vi "reinitialize pico.vi"(8 "error in (no error)":errorcluster, 11 "Picomotor8742dotNet in":refnum<class "Picomotor8742dotNet.lvclass">) -> (0 "error out":errorcluster, 2 "new command":string, 3 "Picomotor8742dotNet out":refnum<class "Picomotor8742dotNet.lvclass">)   [LabVIEW 2020, in "Picomotor8742dotNet.lvclass"]
uses:
  Picomotor8742dotNet.lvclass
  Picomotor8742dotNet.lvclass/Picomotor8742dotNet.ctl
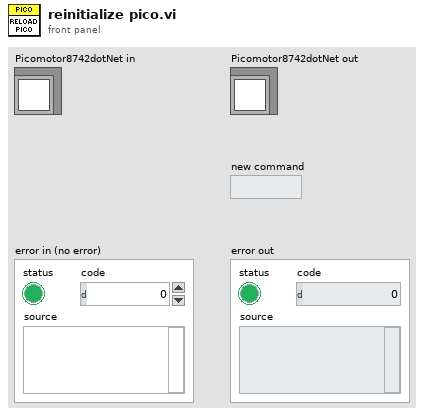
[diagram p1: front panel]
types:
  T1 = typedef "Picomotor8742dotNet.lvclass/Settings_Typdef.ctl" = cluster{"Position":cluster{"Axis 1":cluster{"Value":dbl, "Min":dbl, "Max":dbl, "StepSize":dbl, "Tolerance":dbl, "ValueActual":dbl}, "Axis 2":cluster{"Value":dbl, "Min":dbl, "Max":dbl, "StepSize":dbl, "Tolerance":dbl, "ValueActual":dbl}, "Axis 3":cluster{"Value":dbl, "Min":dbl, "Max":dbl, "StepSize":dbl, "Tolerance":dbl, "ValueActual":dbl}, "Axis 4":cluster{"Value":dbl, "Min":dbl, "Max":dbl, "StepSize":dbl, "Tolerance":dbl, "ValueActual":dbl}}, "ipaddress":string, "Simulation":enum16{"off", "on"}}
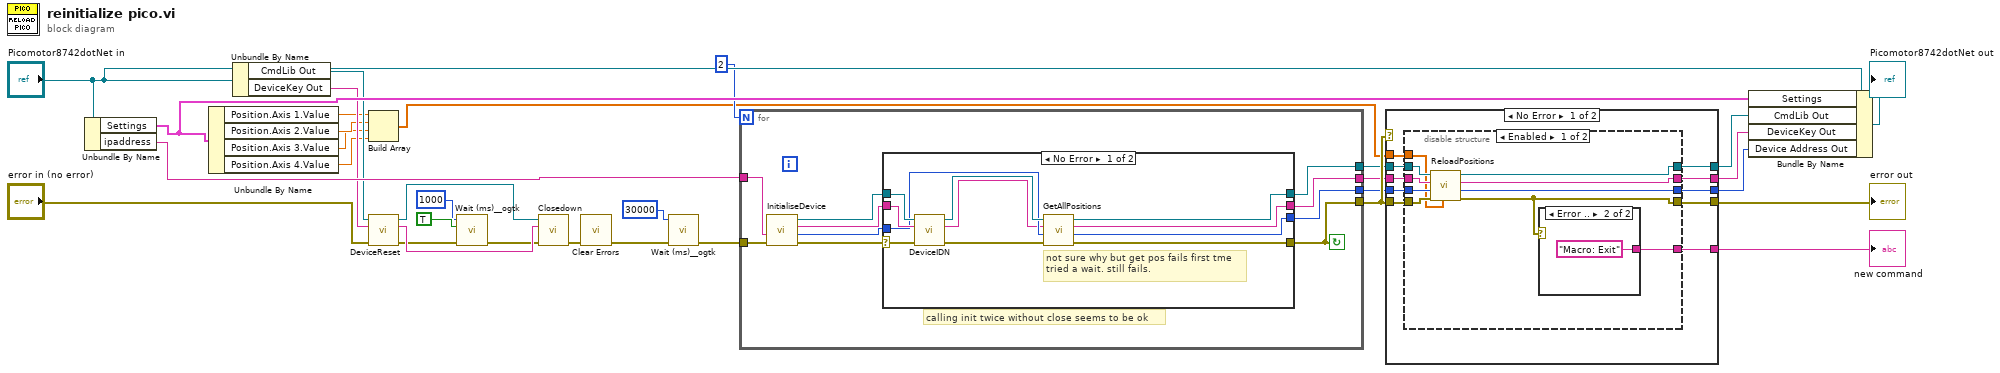
[diagram p0: block diagram]
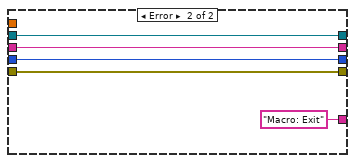
[diagram p4: hidden frame]
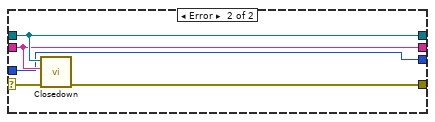
[diagram p5: hidden frame]
diagram:
  n1 = Unbundle By Name("Picomotor8742dotNet in") -> ("Settings"=w31:T1, "ipaddress"=w32:string)
  n2 = Unbundle By Name(w31) -> ("Position.Axis 1.Value"=w8:dbl, "Position.Axis 2.Value"=w11:dbl, "Position.Axis 3.Value"=w10:dbl, "Position.Axis 4.Value"=w9:dbl)
  n3 = Unbundle By Name("Picomotor8742dotNet in") -> ("CmdLib Out"=w21:refnum<k24>, "DeviceKey Out"=w22:string)
  n4 = Build Array(w8, w11, w10, w9) -> (w12:dbl[])
  n5 = call "DeviceReset.vi"("error in (no error)"="error in (no error)", "DeviceKey In"=w22, "CmdLib In"=w21) -> ("error out"=w24:errorcluster, "DeviceKey Out"=w26:string, "CmdLib Out"=w25:refnum<k24>)  [unwired: 2 in]
  n6 = call "Wait (ms)__ogtk.vi"("error in (no error)"=w24, "Wait on Error (FALSE)"=TRUE, "milliseconds to wait"=u32 1000) -> ("error out"=w16:errorcluster)  [unwired: 7 in, 1 out]
  n7 = call "Closedown.vi"("error In"=w16, "DeviceKey In"=w26, "CmdLib In"=w25) -> ("error out"=w17:errorcluster)  [unwired: 8 in]
  n8 = call "Clear Errors.vi"("error in (no error)"=w17) -> ("error out"=w18:errorcluster)  [unwired: 5 in, 1 out]
  n9 = call "Wait (ms)__ogtk.vi"("error in (no error)"=w18, "milliseconds to wait"=u32 30000) -> ("error out"=w19:errorcluster)  [unwired: 8 in, 1 out]
  n10 = for {
    N: 2 -> [_]
    tunnel: [w36] -> w2
    tunnel: [w33] -> w4
    tunnel: w19 -> [w41]
    tunnel: [w37] -> w29
    tunnel: w32 -> [w42]
    tunnel: [w35] -> w3
    stop <- w37 continue-if-true
    # "calling init twice without close seems to be ok"
    n11 = call "InitialiseDevice.vi"("error In"=w41, "PicoMotor IP In"=w42) -> ("error out"=w39:errorcluster, "DreviceAddressOut"=w34:i32, "DeviceKey Out"=w38:string, "CmdLib Out"=w40:refnum<k24>)  [unwired: 6 in]
    n12 = case shown="No Error" w39 {
      selector: w39 -> [w53 w57]
      tunnel: w40 -> [w51 w56]
      tunnel: w38 -> [w52 w55]
      tunnel: [w50 w58] -> w37
      tunnel: [w44 w56] -> w36
      tunnel: [w45 w55] -> w35
      tunnel: w34 -> [w48 w54]
      tunnel: [w47 w54] -> w33
      frame No Error {
        # "not sure why but get pos fails first tme\ntried a wait. still fails."
        n13 = call "DeviceIDN.vi"("error in (no error)"=w53, "DeviceKey In"=w52, "CmdLib In"=w51) -> ("error out"=w43:errorcluster, "DeviceKey Out"=w46:string, "CmdLib Out"=w49:refnum<k24>)  [unwired: 1 in, 1 out]
        n14 = call "GetAllPositions.vi"("error In"=w43, "Device Address In"=w48, "DeviceKey In"=w46, "CmdLib In"=w49) -> ("error out"=w50:errorcluster, "Device Address Out"=w47:i32, "DeviceKey Out"=w45:string, "CmdLib Out"=w44:refnum<k24>)  [unwired: 3 in, 1 out]
      }
      frame Error {
        n15 = call "Closedown.vi"("error In"=w57, "DeviceKey In"=w55, "CmdLib In"=w56) -> ("error out"=w58:errorcluster)  [unwired: 8 in]
      }
    }
  }
  n16 = case shown="No Error" w29 {
    tunnel: w2 -> [w68 w87]
    tunnel: w3 -> [w67 w88]
    tunnel: w4 -> [w66 w86]
    tunnel: w29 -> [w65 w85]
    tunnel: [w64 w87] -> w5
    tunnel: [w63 w88] -> w6
    tunnel: [w62 w86] -> w7
    tunnel: w12 -> [w61 _]
    tunnel: [w60 w85] -> w13
    tunnel: [w59 "Macro: Exit" ("new command")] -> w28
    frame No Error {
      n17 = disable-structure shown="Enabled" {
        disable-tunnel: w68 -> [w78 w83]
        disable-tunnel: w67 -> [w77 w82]
        disable-tunnel: w66 -> [w76 w81]
        disable-tunnel: w65 -> [w75 w80]
        disable-tunnel: [w74 w83] -> w64
        disable-tunnel: [w73 w82] -> w63
        disable-tunnel: [w72 w81] -> w62
        disable-tunnel: w61 -> [w71 _]
        disable-tunnel: [w70 w80] -> w60
        disable-tunnel: [w69 _] -> w59
        frame Enabled {
          n18 = call "ReloadPositions.vi"("Load Positions"=w71, "error In"=w75, "Device Address In"=w76, "DeviceKey In"=w77, "CmdLib In"=w78) -> ("error Out"=w70:errorcluster, "Device Address Out"=w72:i32, "DeviceKey Out"=w73:string, "CmdLib Out"=w74:refnum<k24>)  [unwired: 3 in]
          n19 = case shown="Error .." w70 {
            tunnel: [_ "Macro: Exit" ("new command")] -> w69
            frame No Error {
            }
            frame Error {
            }
          }
        }
        frame Disabled {
        }
      }
    }
    frame Error {
    }
  }
  "new command" <- w28
  "error out" <- w13
  n20 = Bundle By Name(cluster="Picomotor8742dotNet in", "Settings"=w31, "CmdLib Out"=w5, "DeviceKey Out"=w6, "Device Address Out"=w7) -> (→"Picomotor8742dotNet out":refnum<class "Picomotor8742dotNet.lvclass">)
